vi "Write Trigger Frequency.vi"(8 "error in (no error)":errorcluster, 10 "Trigger Frequency":dbl, 11 "Galvo in":refnum<class "Galvo.lvclass">) -> (0 "error out":errorcluster, 3 "Galvo out":refnum<class "Galvo.lvclass">)   [LabVIEW 2015, in "Galvo.lvclass"]
uses:
  Galvo.lvclass
  Galvo.lvclass/Galvo.ctl
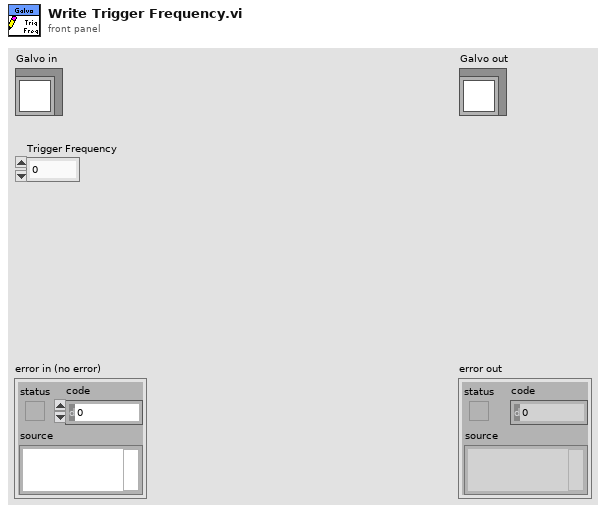
[diagram p1: front panel]
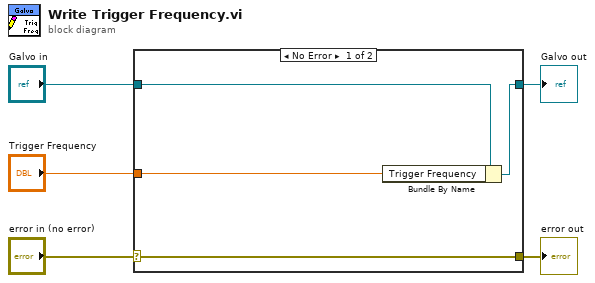
[diagram p0: block diagram]
diagram:
  n1 = case shown="No Error" "error in (no error)" {
    selector: "error in (no error)" -> [w9 w10]
    tunnel: [w9 w10] -> w4
    tunnel: [w7 w11] -> w2
    tunnel: "Galvo in" -> [w8 w11]
    tunnel: "Trigger Frequency" -> [w6 _]
    frame No Error {
      n2 = Bundle By Name(cluster=w8, "Trigger Frequency"=w6) -> (w7:refnum<class "Galvo.lvclass">)
    }
    frame Error {
    }
  }
  "error out" <- w4
  "Galvo out" <- w2
